vi "Test sqlite3.vi"() -> ()   [LabVIEW 2020]
uses:
  externals/sqlite3/Source/sqlite3.lvclass/sqlite3.ctl
  <vilib>/Utility/error.llb/Error Cluster From Error Code.vi
  externals/sqlite3/Source/sqlite3.lvclass
panel:
  in  "value":string="value123"
  out "Result":string
  out "error out":errorcluster
  in  "DatabaseFilePath":path
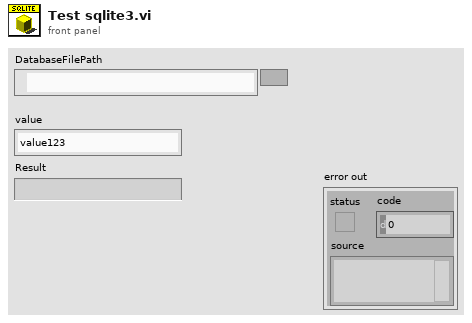
[diagram p1: front panel]
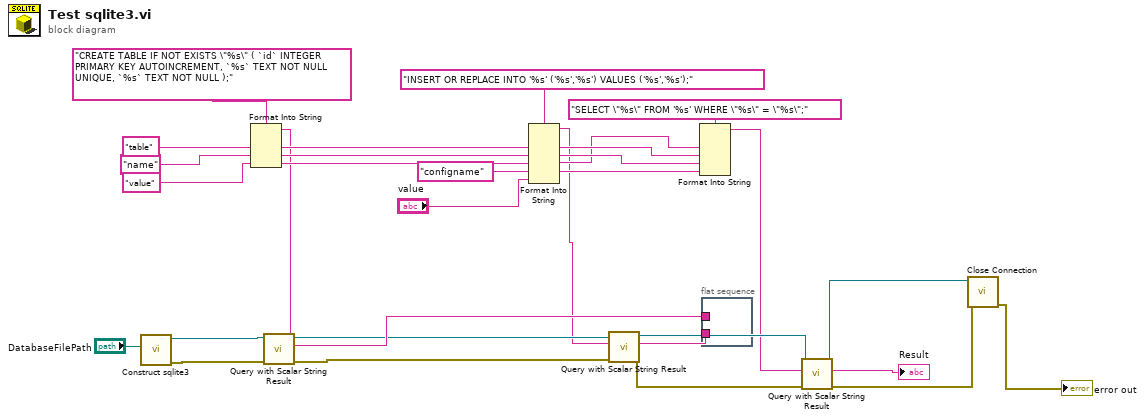
[diagram p0: block diagram]
diagram:
  w18 = "configname" ("input 4")
  w16 = "value" ("input 3")
  w19 = "name" ("input 2")
  w17 = "table"
  n1 = call "Construct sqlite3.vi"("DatabaseFilePath"="DatabaseFilePath") -> ("error out"=w14:errorcluster, "sqlite3 out"=w15:refnum<class "sqlite3.lvclass">)  [unwired: 9 in]
  n2 = Format Into String(format string="CREATE TABLE IF NOT EXISTS \"%s\" ( `id` INTEGER PRIMARY KEY AUTOINCREMENT, `%s` TEXT NOT NULL UNIQUE, `%s` TEXT NOT NULL );" ("Query out 2"), w17, w19, w16) -> (resulting string=w13:string)  [unwired: 2 in, 1 out]
  n3 = call-dynamic "Query with Scalar String Result.vi"("error in (no error)"=w14, "Query string"=w13, "sqlite3 in"=w15) -> ("error out"=w9:errorcluster, "Result"=w12:string, "sqlite3 out"=w11:refnum<class "sqlite3.lvclass">)  [unwired: 6 in]
  n4 = Format Into String(format string="INSERT OR REPLACE INTO '%s' ('%s','%s') VALUES ('%s','%s');", w17, w19, w16, w18, "value") -> (resulting string=w10:string)  [unwired: 2 in, 1 out]
  n5 = call-dynamic "Query with Scalar String Result.vi"("error in (no error)"=w9, "Query string"=w10, "sqlite3 in"=w11) -> ("error out"=w6:errorcluster, "Result"=w8:string, "sqlite3 out"=w7:refnum<class "sqlite3.lvclass">)  [unwired: 6 in]
  n6 = Format Into String(format string="SELECT \"%s\" FROM '%s' WHERE \"%s\" = \"%s\";", w16, w17, w19, w18) -> (resulting string=w5:string)  [unwired: 2 in, 1 out]
  n7 = flat-sequence {
    tunnel: w12 -> [_]
    tunnel: w8 -> [_]
    frame #0 {
    }
  }
  n8 = call-dynamic "Query with Scalar String Result.vi"("error in (no error)"=w6, "Query string"=w5, "sqlite3 in"=w7) -> ("error out"=w2:errorcluster, "Result"=→"Result":string, "sqlite3 out"=w3:refnum<class "sqlite3.lvclass">)  [unwired: 6 in]
  n9 = call-dynamic "Close Connection.vi"("error in (no error)"=w2, "sqlite in"=w3) -> ("error out"=→"error out":errorcluster)  [unwired: 8 in, 1 out]
